vi "NI DOCO DEMO_Different Sample.vi"() -> ()   [LabVIEW 2018]
uses:
  <vilib>/DAQmx/write.llb/DAQmx Write (Digital 1D Wfm NChan NSamp).vi
  <vilib>/DAQmx/write.llb/DAQmx Write (Analog 1D Wfm NChan NSamp).vi
  <vilib>/DAQmx/create/channels.llb/DAQmx Create Channel (AO-Voltage-Basic).vi
  <vilib>/DAQmx/configure/timing.llb/DAQmx Timing (Sample Clock).vi
  <vilib>/Waveform/WDTOps.llb/WDT Number of Waveform Samples DBL.vi
  <vilib>/Waveform/WDTOps.llb/WDT Append Waveforms DBL.vi
  <vilib>/DAQmx/miscellaneous.llb/DAQmx Fill In Error Info.vi
  <vilib>/Waveform/DTblOps.llb/DTbl Digital to Boolean Array.vi
  <vilib>/DAQmx/create/channels.llb/DAQmx Create Channel (DO-Digital Output).vi
  <vilib>/Waveform/DWDTOps.llb/DWDT Uncompress Digital.vi
  <vilib>/Waveform/DWDTOps.llb/DWDT Append Digital Samples.vi
  <resource>/objmgr/daqmx.rc
panel:
  out "number of samples 4":i32
  out "element":i32
  out "size(s) 3":i32
  out "Mixed Signal Graph 3":cluster{digitalwaveform[]}(graph)
  out "Numeric 2":u32
  out "DO size 3":i32
  out "DO size 2":i32
  out "DO size":i32
  out "number of samples 3":i32
  out "number of samples 2":i32
  out "number of samples":i32
  out "Mixed Signal Graph 2":cluster{waveform(dbl)[]}(graph)
  out "Mixed Signal Graph":cluster{waveform(dbl)[], digitalwaveform[]}(graph)
  out "initialized array":digitalwaveform[](array[waveform])
  out "Waveform Graph":waveform(dbl)[](graph)=[{"t0"=timestamp(0 s since 1904-01-01), "dt"=2e-05, "Y"=array[34500 elements]}, {"t0"=timestamp(0 s since 1904-01-01), "dt"=2e-05, "Y"=array[34500 elements]}, {"t0"=timestamp(0 s since 1904-01-01), "dt"=2e-05, "Y"=array[34500 elements]}, {"t0"=timestamp(0 s since 1904-01-01), "dt"=2e-05, "Y"=array[34500 elements]}, {"t0"=timestamp(0 s since 1904-01-01), "dt"=2e-05, "Y"=array[34500 elements]}, {"t0"=timestamp(0 s since 1904-01-01), "dt"=2e-05, "Y"=array[34500 elements]}, {"t0"=timestamp(0 s since 1904-01-01), "dt"=2e-05, "Y"=array[34500 elements]}, {"t0"=timestamp(0 s since 1904-01-01), "dt"=2e-05, "Y"=array[34500 elements]}]
  out "Digital Waveform Graph":digitalwaveform[](graph)
  out "size(s) 4":i32
  out "size(s) 2":i32
  out "size(s)":i32
  out "NumChans 2":u32
  out "NumChans":u32
  out "Numeric":u32
  in  "Enum":enum16{"A A", "A B", "B B", "B A"}(ring)
  in  "stop 2":bool
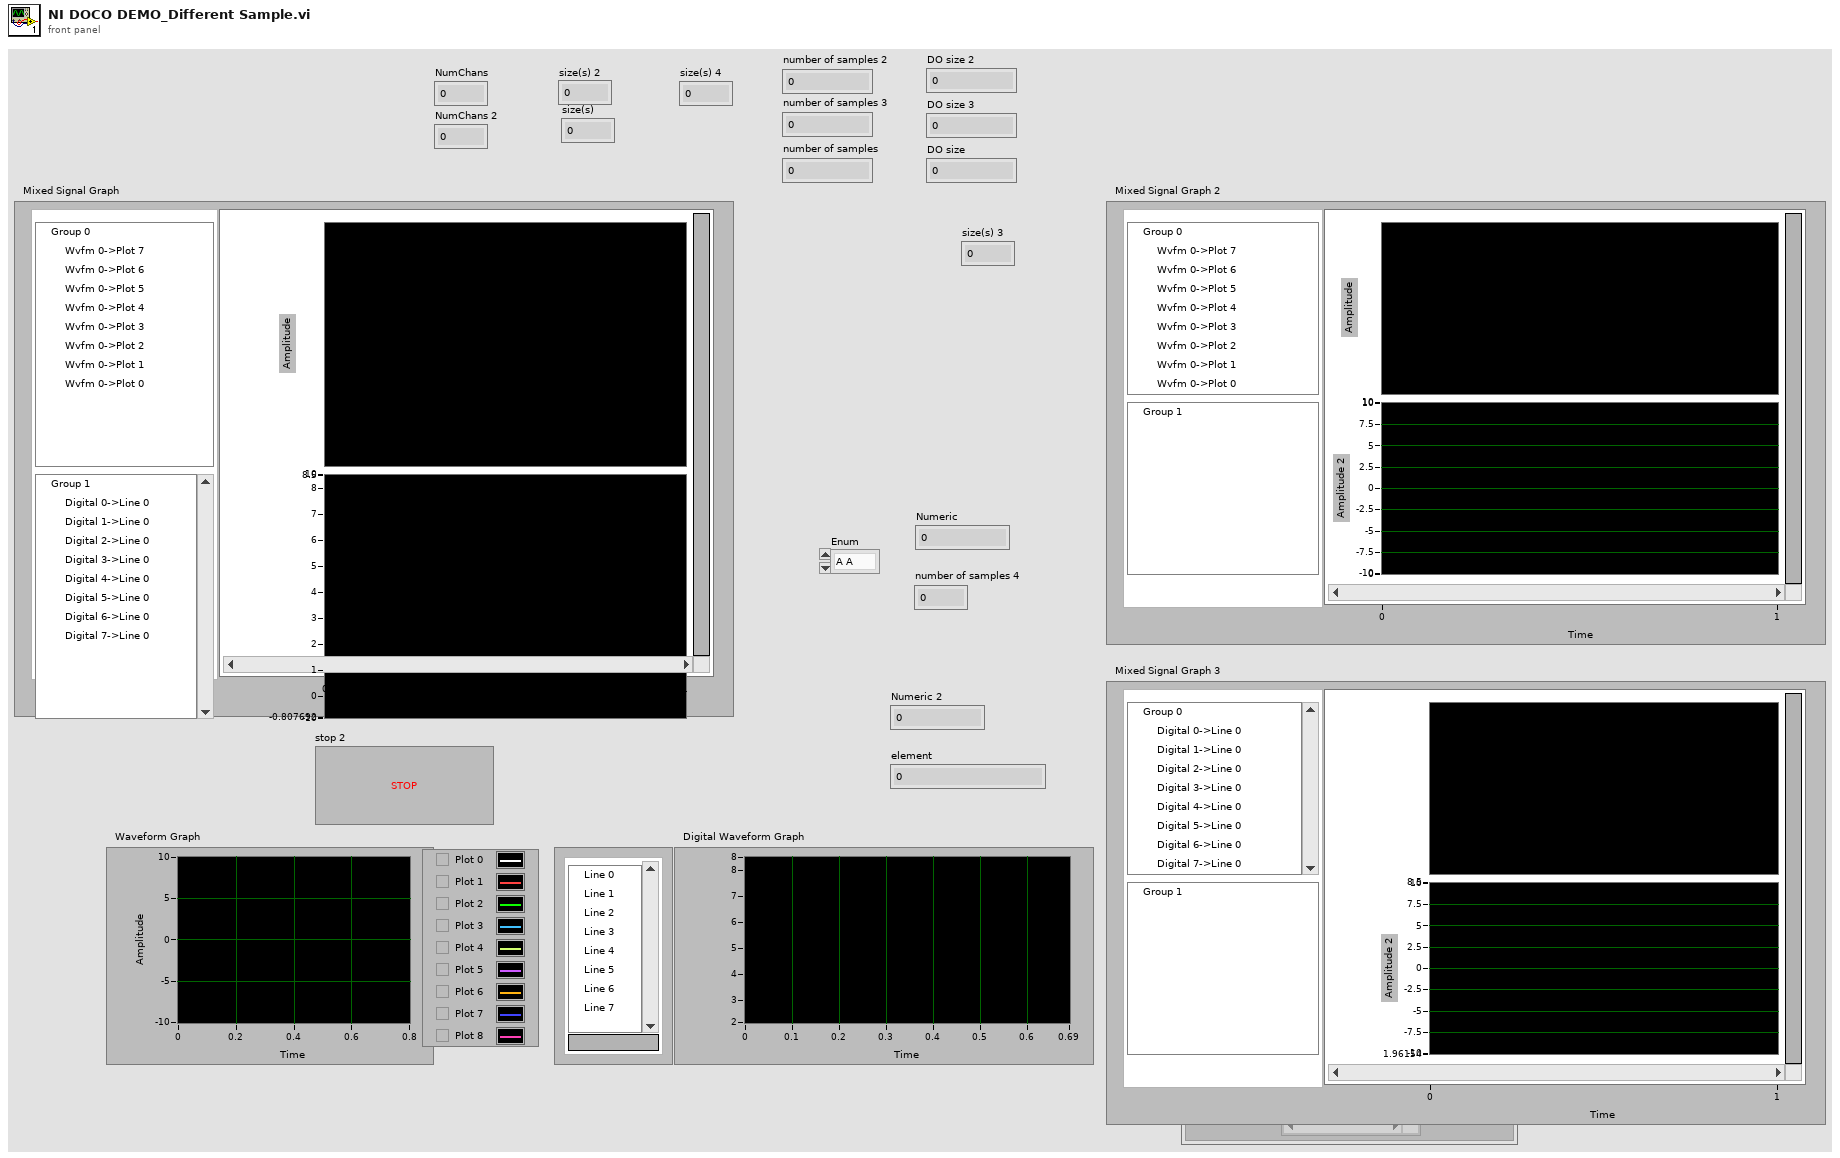
[diagram p1: front panel]
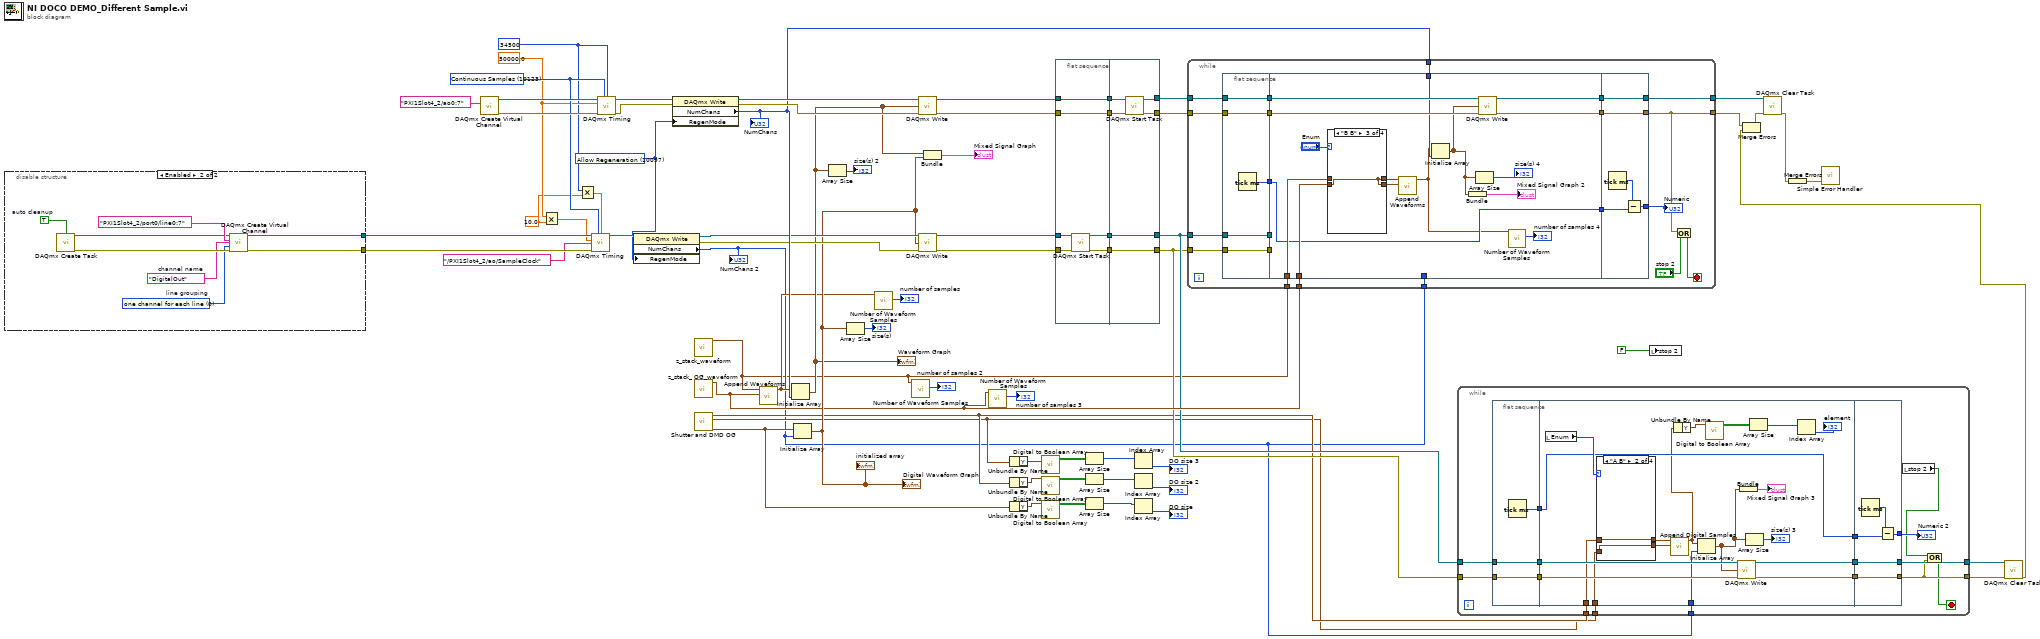
[diagram p0: block diagram]
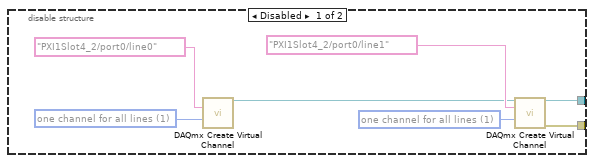
[diagram p5: hidden frame]
diagram:
  w1 = 10.0 ("y")
  w37 = 10097 items=["Allow Regeneration"=10097, "Do Not Allow Regeneration"=10158] ("RegenMode")
  w35 = 34500 ("samples per channel")
  w64 = 10123 items=["Finite Samples"=10178, "Continuous Samples"=10123, "Hardware Timed Single Point"=12522] ("sample mode")
  w36 = 50000.0 ("rate")
  n1 = disable-structure shown="Enabled" {
    disable-tunnel: [w75 w77] -> w66
    disable-tunnel: [w74 w78] -> w65
    frame Disabled {
      w70 = 1 items=["one channel for each line", "one channel for all lines"] ("line grouping")
      w73 = 1 items=["one channel for each line", "one channel for all lines"] ("line grouping")
      n2 = call-poly <vilib>:"DAQmx Create Virtual Channel.vi"("lines"=tag "PXI1Slot4_2/port0/line0", "line grouping"=w70) -> ("task out"=w71:refnum<k21>)  [unwired: 12 in, 1 out]
      n3 = call-poly <vilib>:"DAQmx Create Virtual Channel.vi"("task in"=w71, "lines"=tag "PXI1Slot4_2/port0/line1", "line grouping"=w73) -> ("task out"=w74:refnum<k21>, "error out"=w75:errorcluster)  [unwired: 11 in]
    }
    frame Enabled {
      w79 = TRUE  # auto cleanup
      w83 = 0 items=["one channel for each line", "one channel for all lines"]  # line grouping
      w82 = "DigitalOut"  # channel name
      n4 = call <vilib>:"DAQmx Create Task.vi"("auto cleanup"=w79) -> ("task out"=w80:refnum<k21>, "error out"=w84:errorcluster)  [unwired: 13 in]
      n5 = call-poly <vilib>:"DAQmx Create Virtual Channel.vi"("task in"=w80, "lines"=tag "PXI1Slot4_2/port0/line0:7", "name to assign"=w82, "line grouping"=w83, "error in"=w84) -> ("task out"=w78:refnum<k21>, "error out"=w77:errorcluster)  [unwired: 9 in]
    }
  }
  n6 = call-poly <vilib>:"DAQmx Create Virtual Channel.vi"("physical channels"=tag "PXI1Slot4_2/ao0:7") -> ("task out"=w68:refnum<k21>, "error out"=w67:errorcluster)  [unwired: 13 in]
  n7 = Multiply(x=w36, y=w1) -> (x*y=w2:dbl)
  n8 = Multiply(x=w35, y=w1) -> (x*y=w34:dbl)
  n9 = call-poly <vilib>:"DAQmx Timing.vi"("task/channels in"=w65, "sample mode"=w64, "samples per channel"=w34, "rate"=w2, "source"=tag "/PXI1Slot4_2/ao/SampleClock", "error in"=w66) -> ("task out"=w44:refnum<k21>)  [unwired: 8 in, 1 out]
  n10 = call-poly <vilib>:"DAQmx Timing.vi"("task/channels in"=w68, "sample mode"=w64, "samples per channel"=w35, "rate"=w36, "error in"=w67) -> ("task out"=w49:refnum<k21>, "error out"=w48:errorcluster)  [unwired: 9 in]
  n11 = property class="DAQmx Write"(reference=w44, "RegenMode"=w37) -> (reference out=w43:refnum<k21>, error out=w42:errorcluster, "NumChans"=w5:u32)  [unwired: 1 in]
  "NumChans 2" <- w5
  n12 = property class="DAQmx Write"(reference=w49, error in=w48, "RegenMode"=w37) -> (reference out=w47:refnum<k21>, error out=w46:errorcluster, "NumChans"=w45:u32)
  "NumChans" <- w45
  n13 = call "z_stack_waveform.vi"() -> ("waveform out"=w3:waveform(dbl))  [unwired: 9 in, 2 out]
  n14 = call "z_stack_ OG_waveform.vi"() -> ("waveform out"=w29:waveform(dbl))  [unwired: 15 in, 4 out]
  n15 = call "Shutter and DMD OG.vi"() -> ("output waveform"=w27:digitalwaveform, "output waveform 2"=w11:digitalwaveform, "output waveform1"=w12:digitalwaveform)  [unwired: 8 in]
  n16 = call-poly <vilib>:"Append Waveforms.vi"("waveform B"=w29, "waveform A"=w3) -> ("waveform out"=w31:waveform(dbl))  [unwired: 8 in, 1 out]
  n17 = Initialize Array(w31, w45) -> (w33:waveform(dbl)[])
  "Waveform Graph" <- w33
  n18 = Initialize Array(w27, w5) -> (w39:digitalwaveform[])
  "Digital Waveform Graph" <- w39
  "initialized array" <- w39
  n19 = Array Size(array=w33) -> (size(s)=→"size(s) 2":i32)
  n20 = Array Size(array=w39) -> (size(s)=→"size(s)":i32)
  n21 = call-poly <vilib>:"Number of Waveform Samples.vi"("waveform in"=w31) -> ("number of samples"=→"number of samples":i32)  [unwired: 8 in, 2 out]
  n22 = call-poly <vilib>:"Number of Waveform Samples.vi"("waveform in"=w3) -> ("number of samples"=→"number of samples 2":i32)  [unwired: 8 in, 2 out]
  n23 = call-poly <vilib>:"DAQmx Write.vi"("task/channels in"=w47, "data"=w33, "error in"=w46) -> ("task out"=w62:refnum<k21>, "error out"=w58:errorcluster)  [unwired: 10 in, 1 out]
  n24 = call-poly <vilib>:"DAQmx Write.vi"("task/channels in"=w43, "data"=w39, "error in"=w42) -> ("task out"=w51:refnum<k21>, "error out"=w50:errorcluster)  [unwired: 10 in, 1 out]
  n25 = Bundle(w33, w39) -> (→"Mixed Signal Graph":cluster{waveform(dbl)[], digitalwaveform[]})  [unwired: 1 in]
  n26 = call-poly <vilib>:"Number of Waveform Samples.vi"("waveform in"=w29) -> ("number of samples"=→"number of samples 3":i32)  [unwired: 8 in, 2 out]
  n27 = Unbundle By Name(w11) -> ("Y"=w21:digitaldata)
  n28 = Unbundle By Name(w12) -> ("Y"=w19:digitaldata)
  n29 = Unbundle By Name(w27) -> ("Y"=w22:digitaldata)
  n30 = call-poly <vilib>:"Digital to Boolean Array.vi"("digital data"=w21) -> ("boolean array"=w18:bool[][])  [unwired: 9 in, 1 out]
  n31 = call-poly <vilib>:"Digital to Boolean Array.vi"("digital data"=w19) -> ("boolean array"=w17:bool[][])  [unwired: 9 in, 1 out]
  n32 = call-poly <vilib>:"Digital to Boolean Array.vi"("digital data"=w22) -> ("boolean array"=w26:bool[][])  [unwired: 9 in, 1 out]
  n33 = flat-sequence {
    tunnel: w62 -> [w90]
    tunnel: w51 -> [w89]
    tunnel: w50 -> [w88]
    tunnel: [w90] -> w61
    tunnel: [w87] -> w60
    tunnel: [w86] -> w59
    tunnel: w58 -> [w85]
    tunnel: [w85] -> w57
    tunnel: w61 -> [w94]
    tunnel: [w96] -> w14
    tunnel: w60 -> [w96]
    tunnel: [w95] -> w13
    tunnel: w59 -> [w95]
    tunnel: [w93] -> w56
    tunnel: w57 -> [w92]
    tunnel: [w91] -> w55
    frame #0 {
      n34 = call <vilib>:"DAQmx Start Task.vi"("task/channels in"=w89, "error in"=w88) -> ("task out"=w87:refnum<k21>, "error out"=w86:errorcluster)  [unwired: 12 in]
    }
    frame #1 {
      n35 = call <vilib>:"DAQmx Start Task.vi"("task/channels in"=w94, "error in"=w92) -> ("task out"=w93:refnum<k21>, "error out"=w91:errorcluster)  [unwired: 12 in]
    }
  }
  n36 = Array Size(array=w18) -> (size(s)=w16:i32[])
  n37 = Array Size(array=w17) -> (size(s)=w15:i32[])
  n38 = Array Size(array=w26) -> (size(s)=w25:i32[])
  n39 = Index Array(array=w16) -> (element=→"DO size 3":i32)  [unwired: 1 in]
  n40 = Index Array(array=w15) -> (element=→"DO size 2":i32)  [unwired: 1 in]
  n41 = Index Array(array=w25) -> (element=→"DO size":i32)  [unwired: 1 in]
  n42 = while {
    tunnel: w56 -> [w115]
    tunnel: w55 -> [w114]
    tunnel: w14 -> [w117]
    tunnel: w13 -> [w116]
    tunnel: [w112] -> w7
    tunnel: [w113] -> w54
    tunnel: w3 -> [w110]
    tunnel: w29 -> [w109]
    tunnel: w45 -> [w100]
    tunnel: w5 -> [w99]
    stop <- w111 stop-if-true
    n43 = flat-sequence {
      tunnel: w114 -> [w119]
      tunnel: w115 -> [w120]
      tunnel: w116 -> [w121]
      tunnel: w117 -> [w122]
      tunnel: [w122] -> w108
      tunnel: [w121] -> w107
      tunnel: [w120] -> w106
      tunnel: [w119] -> w105
      tunnel: [w118] -> w102
      tunnel: w110 -> [w133]
      tunnel: w109 -> [w132]
      tunnel: w108 -> [_]
      tunnel: w107 -> [_]
      tunnel: w106 -> [w138]
      tunnel: w105 -> [w137]
      tunnel: [w136] -> w104
      tunnel: [w135] -> w103
      tunnel: w102 -> [w125]
      tunnel: w100 -> [w129]
      tunnel: w99 -> [_]
      tunnel: [w125] -> w98
      tunnel: [w148] -> w112
      tunnel: [w149] -> w113
      tunnel: w104 -> [w149]
      tunnel: w103 -> [w148]
      tunnel: [w146] -> w101
      tunnel: w98 -> [w145]
      frame #0 {
        n44 = Tick Count (ms)() -> (millisecond timer value=w118:u32)
      }
      frame #1 {
        n45 = case shown="\"B B\"" "Enum" {
          tunnel: w133 -> [w139 w141 _ w143]
          tunnel: w132 -> [_ w140 w142 w144]
          tunnel: [w139 w141 w142 w144] -> w131
          tunnel: [w139 w140 w142 w143] -> w130
          frame "A A", Default {
          }
          frame "A B" {
          }
          frame "B B" {
          }
          frame "B A" {
          }
        }
        n46 = call-poly <vilib>:"Append Waveforms.vi"("waveform B"=w130, "waveform A"=w131) -> ("waveform out"=w124:waveform(dbl))  [unwired: 8 in, 1 out]
        n47 = Initialize Array(w124, w129) -> (w128:waveform(dbl)[])
        n48 = Bundle(w128) -> (→"Mixed Signal Graph 2":cluster{waveform(dbl)[]})  [unwired: 1 in]
        n49 = Array Size(array=w128) -> (size(s)=→"size(s) 4":i32)
        n50 = call-poly <vilib>:"DAQmx Write.vi"("task/channels in"=w138, "data"=w128, "error in"=w137) -> ("task out"=w136:refnum<k21>, "error out"=w135:errorcluster)  [unwired: 10 in, 1 out]
        n51 = call-poly <vilib>:"Number of Waveform Samples.vi"("waveform in"=w124) -> ("number of samples"=→"number of samples 4":i32)  [unwired: 8 in, 2 out]
      }
      frame #2 {
        n52 = Tick Count (ms)() -> (millisecond timer value=w147:u32)
        n53 = Subtract(x=w147, y=w145) -> (x-y=w146:u32)
      }
    }
    n54 = Compound Arithmetic op=OR(w112, "stop 2") -> (w111:bool)
    "Numeric" <- w101
  }
  n55 = while {
    tunnel: w14 -> [w165]
    tunnel: w13 -> [w164]
    tunnel: [w163] -> w9
    tunnel: [w162] -> w10
    tunnel: w12 -> [w160]
    tunnel: w11 -> [w159]
    tunnel: w5 -> [w151]
    stop <- w161 stop-if-true
    n56 = flat-sequence {
      tunnel: w164 -> [w167]
      tunnel: w165 -> [w168]
      tunnel: [w168] -> w158
      tunnel: [w167] -> w157
      tunnel: [w166] -> w154
      tunnel: w160 -> [w183]
      tunnel: w159 -> [w182]
      tunnel: w158 -> [w187]
      tunnel: w157 -> [w186]
      tunnel: [w185] -> w156
      tunnel: [w184] -> w155
      tunnel: w154 -> [w176]
      tunnel: [w176] -> w152
      tunnel: w151 -> [w175]
      tunnel: [w197] -> w162
      tunnel: [w198] -> w163
      tunnel: w156 -> [w198]
      tunnel: w155 -> [w197]
      tunnel: [w195] -> w153
      tunnel: w152 -> [w194]
      frame #0 {
        n57 = Tick Count (ms)() -> (millisecond timer value=w166:u32)
      }
      frame #1 {
        n58 = local read "Enum"() -> (w177:enum16{"A A", "A B", "B B", "B A"})
        n59 = case shown="\"A B\"" w177 {
          tunnel: w183 -> [w188 w190 _ w192]
          tunnel: w182 -> [_ w189 w191 w193]
          tunnel: [w188 w190 w191 w193] -> w181
          tunnel: [w188 w189 w191 w192] -> w180
          frame "A A", Default {
          }
          frame "A B" {
          }
          frame "B B" {
          }
          frame "B A" {
          }
        }
        n60 = call-poly <vilib>:"Append Digital Samples.vi"("digital waveform B"=w180, "digital waveform A"=w181) -> ("digital waveform out"=w170:digitalwaveform)  [unwired: 8 in, 1 out]
        n61 = Unbundle By Name(w170) -> ("Y"=w171:digitaldata)
        n62 = Initialize Array(w170, w175) -> (w179:digitalwaveform[])
        n63 = call-poly <vilib>:"Digital to Boolean Array.vi"("digital data"=w171) -> ("boolean array"=w173:bool[][])  [unwired: 9 in, 1 out]
        n64 = call-poly <vilib>:"DAQmx Write.vi"("task/channels in"=w187, "data"=w179, "error in"=w186) -> ("task out"=w185:refnum<k21>, "error out"=w184:errorcluster)  [unwired: 10 in, 1 out]
        n65 = Bundle(w179) -> (→"Mixed Signal Graph 3":cluster{digitalwaveform[]})  [unwired: 1 in]
        n66 = Array Size(array=w179) -> (size(s)=→"size(s) 3":i32)
        n67 = Array Size(array=w173) -> (size(s)=w172:i32[])
        n68 = Index Array(array=w172) -> (element=→"element":i32)  [unwired: 1 in]
      }
      frame #2 {
        n69 = Tick Count (ms)() -> (millisecond timer value=w196:u32)
        n70 = Subtract(x=w196, y=w194) -> (x-y=w195:u32)
      }
    }
    n71 = local read "stop 2"() -> (w150:bool)
    n72 = Compound Arithmetic op=OR(w150, w162) -> (w161:bool)
    "Numeric 2" <- w153
  }
  n73 = local write "stop 2"(FALSE ("stop 2")) -> ()
  n74 = call <vilib>:"DAQmx Clear Task.vi"("task in"=w9, "error in"=w10) -> ("error out"=w6:errorcluster)  [unwired: 13 in]
  n75 = Merge Errors(w7, w6) -> (w8:errorcluster)
  n76 = call <vilib>:"DAQmx Clear Task.vi"("task in"=w54, "error in"=w8) -> ("error out"=w53:errorcluster)  [unwired: 13 in]
  n77 = Merge Errors(w53) -> (w52:errorcluster)
  n78 = call <vilib>:"Simple Error Handler.vi"("error in (no error)"=w52) -> ()  [unwired: 4 in, 5 out]
